vi "InitializeSmovement.vi"(8 "error in":errorcluster, 9 "slowMoveParams":T2={"slowMoveWavePts"=1024, "slowMoveAccelPts"=128, "moveSpeedSec"=0.2}, 10 "ioParams":cluster{"outputRateHz":u32}={"outputRateHz"=800000}, 11 "FPGAInterfaceIn":T1) -> (0 "error out":errorcluster, 3 "FPGAInterfaceOut":T1)   [LabVIEW 2016]
uses:
  controls/FPGAVIreferenceTypeDefScanEngine.ctl
  <vilib>/Utility/error.llb/Error Cluster From Error Code.vi
  <vilib>/rvi/errors/niLvFpgaAdjustHostInterfaceError.vi
  <vilib>/rvi/interface/nirviReadWriteControl/nirviReadWriteControl.xnode
  FPGA Bitfiles/qnmController797_usbRIO_controllerFPGAmu.lvbitx
  NiFpgaLv.dll
panel:
  in  "stop":bool
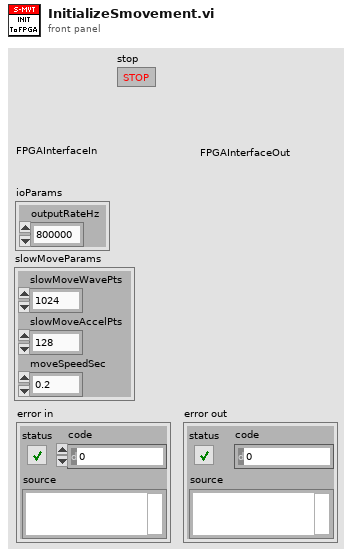
[diagram p1: front panel]
types:
  T1 = typedef "FPGAVIreferenceTypeDefScanEngine.ctl" = refnum<k20>
  T2 = cluster{"slowMoveWavePts":u16, "slowMoveAccelPts":u16, "moveSpeedSec":dbl}
  T3 = cluster{"moveToDecFactor":u16, "moveToWaveSize":u16, "se.mot.p.invDec":fxp<+,16,0>}
  T4 = cluster{"write":bool, "index":u16, "data":fxp<+/-,18,5>}
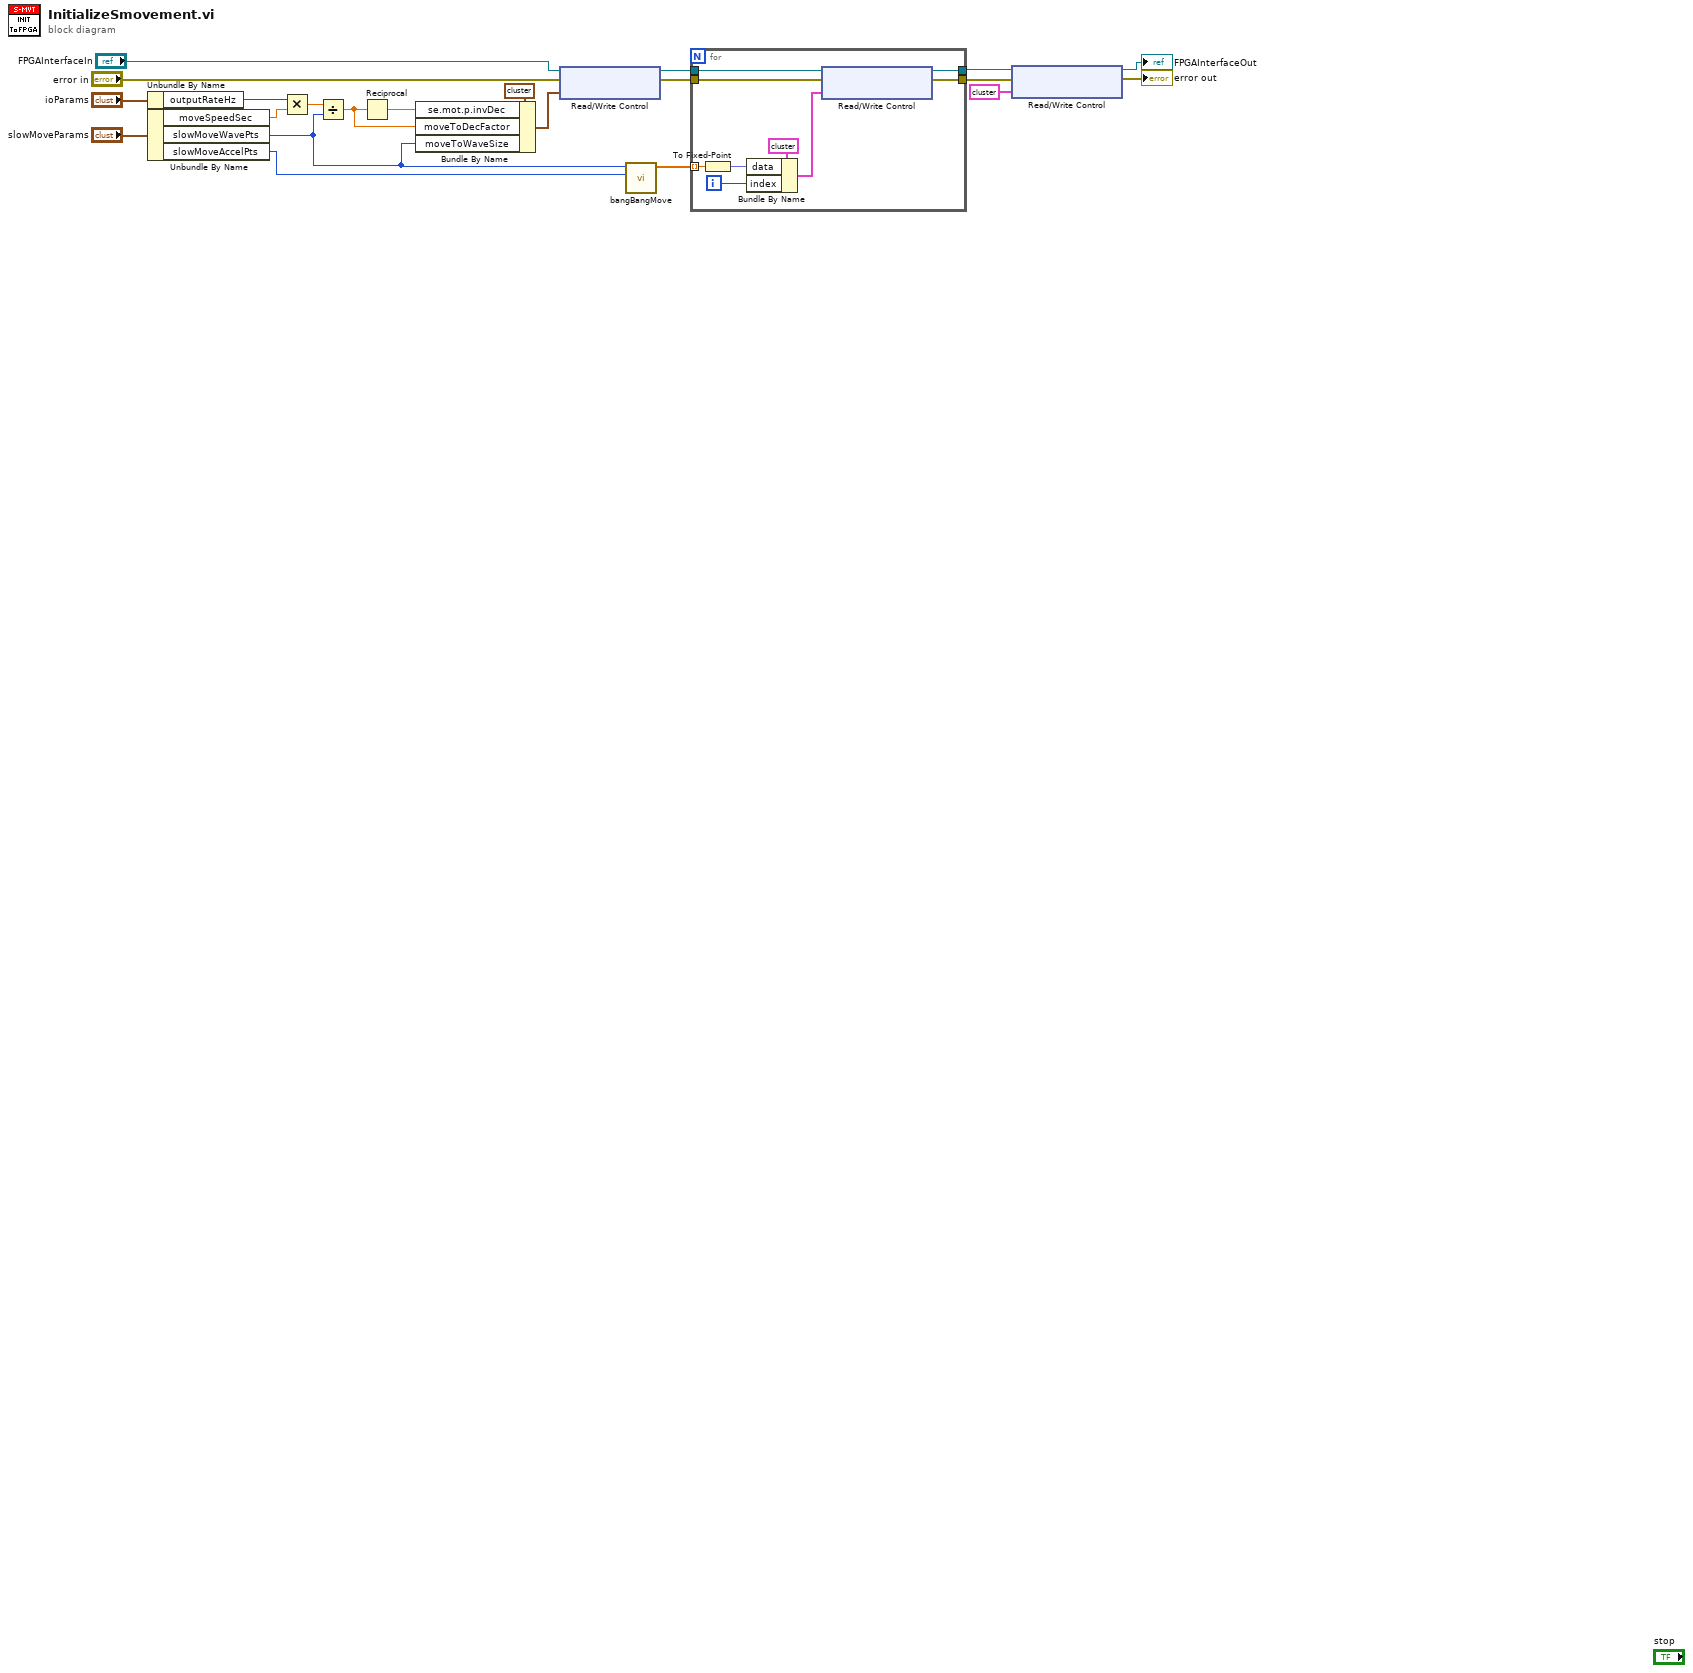
[diagram p0: block diagram]
diagram:
  n1 = Unbundle By Name("ioParams") -> ("outputRateHz"=w17:u32)
  n2 = Unbundle By Name("slowMoveParams") -> ("moveSpeedSec"=w16:dbl, "slowMoveWavePts"=w11:u16, "slowMoveAccelPts"=w20:u16)
  n3 = Multiply(x=w17, y=w16) -> (x*y=w18:dbl)
  n4 = Divide(x=w18, y=w11) -> (x/y=w12:dbl)
  n5 = Reciprocal(x=w12) -> (1/x=w10:dbl)
  n6 = Bundle By Name(cluster=T3 {"moveToDecFactor"=0, "moveToWaveSize"=0, "se.mot.p.invDec"=0.0} ("se.mot.p.clocks"), "se.mot.p.invDec"=w10, "moveToDecFactor"=w12, "moveToWaveSize"=w11) -> (w13:T3)
  n7 = xnode "Read/Write Control"("FPGA VI Reference In"="FPGAInterfaceIn", "error in"="error in", "se.mot.p.clocks"=w13) -> ("FPGA VI Reference Out"=w4:T1, "error out"=w3:errorcluster)
  n8 = call "bangBangMove.vi"("numRoundingPts"=w20, "numPts"=w11) -> ("roundedHalfTriangle"=w19:dbl[])  [unwired: 9 in]
  n9 = for {
    tunnel: w19 -> [w29] mode=indexing
    tunnel: w4 -> [w25]
    tunnel: [w23] -> w6
    tunnel: [w22] -> w7
    tunnel: w3 -> [w26]
    i -> [w30]
    n10 = To Fixed-Point(number=w29) -> (fixed-point=w28:fxp<+/-,18,5>)  [unwired: 1 in]
    n11 = Bundle By Name(cluster=T4 {"write"=TRUE, "index"=0, "data"=0.0} ("moveToWaveWrite"), "data"=w28, "index"=w30) -> (w24:T4)
    n12 = xnode "Read/Write Control"("FPGA VI Reference In"=w25, "error in"=w26, "se.mot.m.motion"=w24) -> ("FPGA VI Reference Out"=w23:T1, "error out"=w22:errorcluster)
  }
  n13 = xnode "Read/Write Control"("FPGA VI Reference In"=w6, "error in"=w7, "se.mot.m.motion"=T4 {"write"=FALSE, "index"=0, "data"=0.0} ("moveToWaveWrite")) -> ("FPGA VI Reference Out"=→"FPGAInterfaceOut":T1, "error out"=→"error out":errorcluster)
